vi "Custom Config.vi"(8 "error in (no error)":errorcluster, 9 "Canon Data":string, 11 "Canon in":refnum<class "Canon.lvclass">) -> (0 "error out":errorcluster, 3 "Canon out":refnum<class "Canon.lvclass">)   [LabVIEW 2021, in "Canon.lvclass"]
uses:
  Canon.lvclass
  Canon.lvclass/Canon.ctl
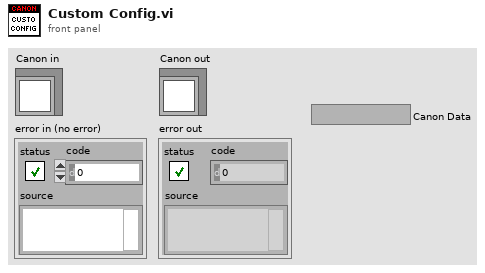
[diagram p1: front panel]
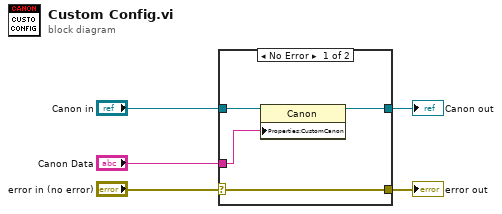
[diagram p0: block diagram]
diagram:
  n1 = case shown="No Error" "error in (no error)" {
    selector: "error in (no error)" -> [w8 w11]
    tunnel: [w8 w11] -> w4
    tunnel: [w7 w10] -> w2
    tunnel: "Canon in" -> [w9 w10]
    tunnel: "Canon Data" -> [w6 _]
    frame No Error {
      n2 = property class="Canon"(reference=w9, "Properties:CustomCanon"=w6) -> (reference out=w7:refnum<class "Canon.lvclass">)  [unwired: 1 in, 1 out]
    }
    frame Error {
    }
  }
  "error out" <- w4
  "Canon out" <- w2
